vi "SGUI Set Variable By Label.vi"(5 "generate error if not found? (True)":bool=TRUE, 7 "value (none)":variant, 10 "error in":errorcluster, 11 "control label (none)":string) -> (2 "error out":errorcluster, 3 "found and type matches?":bool)   [LabVIEW 2013, in "varilib.lvlib"]
doc: "Sets value of any control designated by its label. The reference and label to the control must be first registered by calling 'SGUI Register Controls'. If not found or has invalid type, it will by default return error however it ignores input error (executes anyway). It is up to user to wire a value of a type matching the control data type otherwise it will generate an error."
uses:
  varilib.lvlib
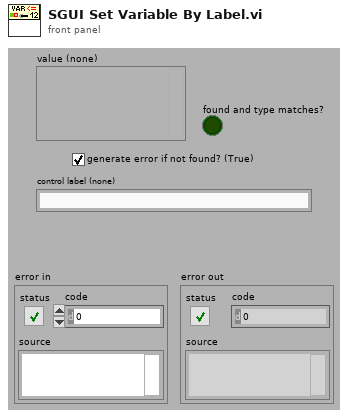
[diagram p1: front panel]
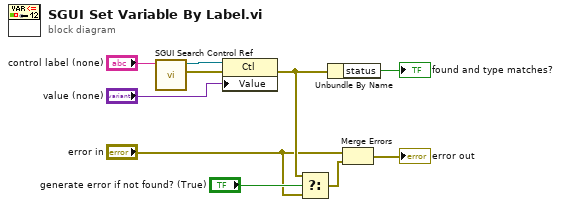
[diagram p0: block diagram]
diagram:
  n1 = call "SGUI Search Control Ref.vi"("control label (empty)"="control label (none)") -> ("error out"=w2:errorcluster, "control ref out"=w1:refnum<vi>)  [unwired: 8 in, 1 out]
  n2 = property class="Ctl"(reference=w1, error in=w2, "Value"="value (none)") -> (error out=w5:errorcluster)  [unwired: 1 out]
  n3 = Select(t=w5, s="generate error if not found? (True)", f="error in") -> (s? t:f=w7:errorcluster)
  n4 = Unbundle By Name(w5) -> ("status"=→"found and type matches?":bool)
  n5 = Merge Errors("error in", w7) -> (→"error out":errorcluster)
